vi "CLIGenerator.vi"(11 "ROS Info":T1={"Node Name"="Node", "Topic Name"="/cmd_lightring", "Message Type"="irobot_create_msgs/msg/LightringLeds", "Message"="{\"override_system\":true,\"leds\":[{\"red\":255,\"green\":0,\"blue\":0},{\"red\":4,\"green\":255,\"blue\":0},{\"red\":6,\"green\":0,\"blue\":255},{\"red\":239,\"green\":142,\"blue\":0},{\"red\":226,\"green\":0,\"blue\":255},{\"red\":0,\"green\":250,\"blue\":255}]}", "Pub_Time"="5"}) -> (3 "CLI":string)   [LabVIEW 2022 SP3]
uses:
  ROSCtrl.ctl
panel:
  # "-1 means \nsubscribe"
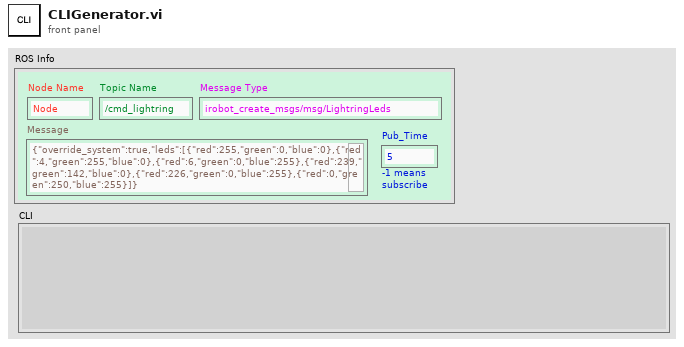
[diagram p1: front panel]
types:
  T1 = typedef "ROSCtrl.ctl" = cluster{"Node Name":string, "Topic Name":string, "Message Type":string, "Message":string, "Pub_Time":string}
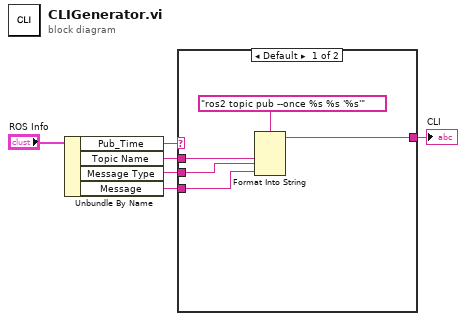
[diagram p0: block diagram]
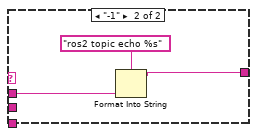
[diagram p2: hidden frame]
diagram:
  n1 = Unbundle By Name("ROS Info") -> ("Pub_Time"=w5:string, "Topic Name"=w4:string, "Message Type"=w3:string, "Message"=w2:string)
  n2 = case shown="Default" w5 {
    tunnel: w4 -> [w10 w14]
    tunnel: w3 -> [w9 _]
    tunnel: w2 -> [w8 _]
    tunnel: [w7 w12] -> w1
    frame Default {
      n3 = Format Into String(format string="ros2 topic pub --once %s %s '%s'", w10, w9, w8) -> (resulting string=w7:string)  [unwired: 2 in, 1 out]
    }
    frame "-1" {
      n4 = Format Into String(format string="ros2 topic echo %s", w14) -> (resulting string=w12:string)  [unwired: 2 in, 1 out]
    }
  }
  "CLI" <- w1
